vi "Unit Test.vi"() -> ()   [LabVIEW 2018]
uses:
  PPLs/Temp Chamber/Parent/Temp Chamber.lvlibp/Custom Controls/Status.ctl
  PPLs/Temp Chamber/Parent/Temp Chamber.lvlibp/Custom Controls/Profile Status.ctl
  PPLs/Temp Chamber/Parent/Temp Chamber.lvlibp/Custom Controls/Profile State.ctl
  PPLs/Temp Chamber/Parent/Temp Chamber.lvlibp/Custom Controls/Step Status.ctl
  PPLs/Temp Chamber/Parent/Temp Chamber.lvlibp/Custom Controls/Step Type.ctl
  F4T.lvclass
  Custom Controls/Command Data.ctl
  PPLs/Temp Chamber/Parent/Temp Chamber.lvlibp/Temp Chamber.lvclass
  PPLs/Temp Chamber/Parent/Temp Chamber.lvlibp/Custom Controls/Control Mode.ctl
  C:/Projects/LabVIEW/PPLs/Temp Chamber/Parent/Temp Chamber.lvlibp/Temp Chamber.lvclass
panel:
  out "Numeric":i32
  out "Value":dbl
  out "Status 2":T1={"Profile Status"={"Profile State"=enum."Not Running", "Current Profile"=0, "Total Time Remaining"=0, "Total Steps"=0}, "Step Status"={"Current Step"=0, "Step Type"=enum."Instant Change", "Time Remaining"=0}}
  out "Status":T1={"Profile Status"={"Profile State"=enum."Not Running", "Current Profile"=0, "Total Time Remaining"=0, "Total Steps"=0}, "Step Status"={"Current Step"=0, "Step Type"=enum."Instant Change", "Time Remaining"=0}}
  in  "reference":refnum<visa-resource-name>="169.254.242.191"
  out "error out":errorcluster
  in  "error in (no error)":errorcluster
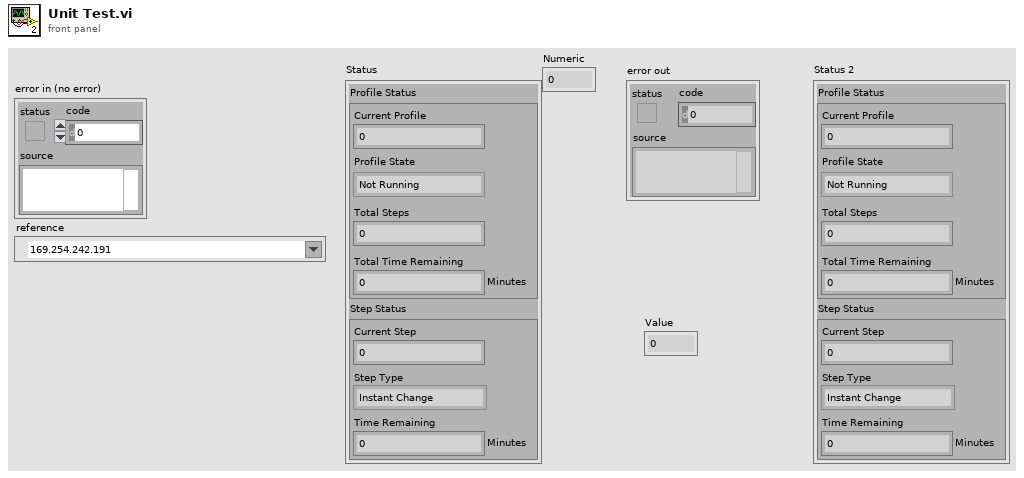
[diagram p1: front panel]
types:
  T1 = typedef "Temp Chamber.lvlibp/Temp Chamber.lvclass/Status.ctl" = cluster{"Profile Status":T2, "Step Status":T4}
  T2 = typedef "Temp Chamber.lvlibp/Temp Chamber.lvclass/Profile Status.ctl" = cluster{"Profile State":T3, "Current Profile":u32, "Total Time Remaining":u32, "Total Steps":u32}
  T3 = typedef "Temp Chamber.lvlibp/Temp Chamber.lvclass/Profile State.ctl" = enum16{"Running", "Not Running", "Paused", "Completed", "Terminated"}
  T4 = typedef "Temp Chamber.lvlibp/Temp Chamber.lvclass/Step Status.ctl" = cluster{"Current Step":u32, "Step Type":T5, "Time Remaining":u32}
  T5 = typedef "Temp Chamber.lvlibp/Temp Chamber.lvclass/Step Type.ctl" = enum16{"Instant Change", "Wait For", "Jump", "Soak", "Ramp Rate", "Ramp Time", "End", "Other"}
  T6 = typedef "F4T.lvlib/F4T.lvclass/Command Data.ctl" = cluster{"ParameterID":u32, "InstanceId":u32, "Value":string}
  T7 = typedef "Temp Chamber.lvlibp/Temp Chamber.lvclass/Control Mode.ctl" = enum16{"Start", "Pause", "Resume", "Stop"}
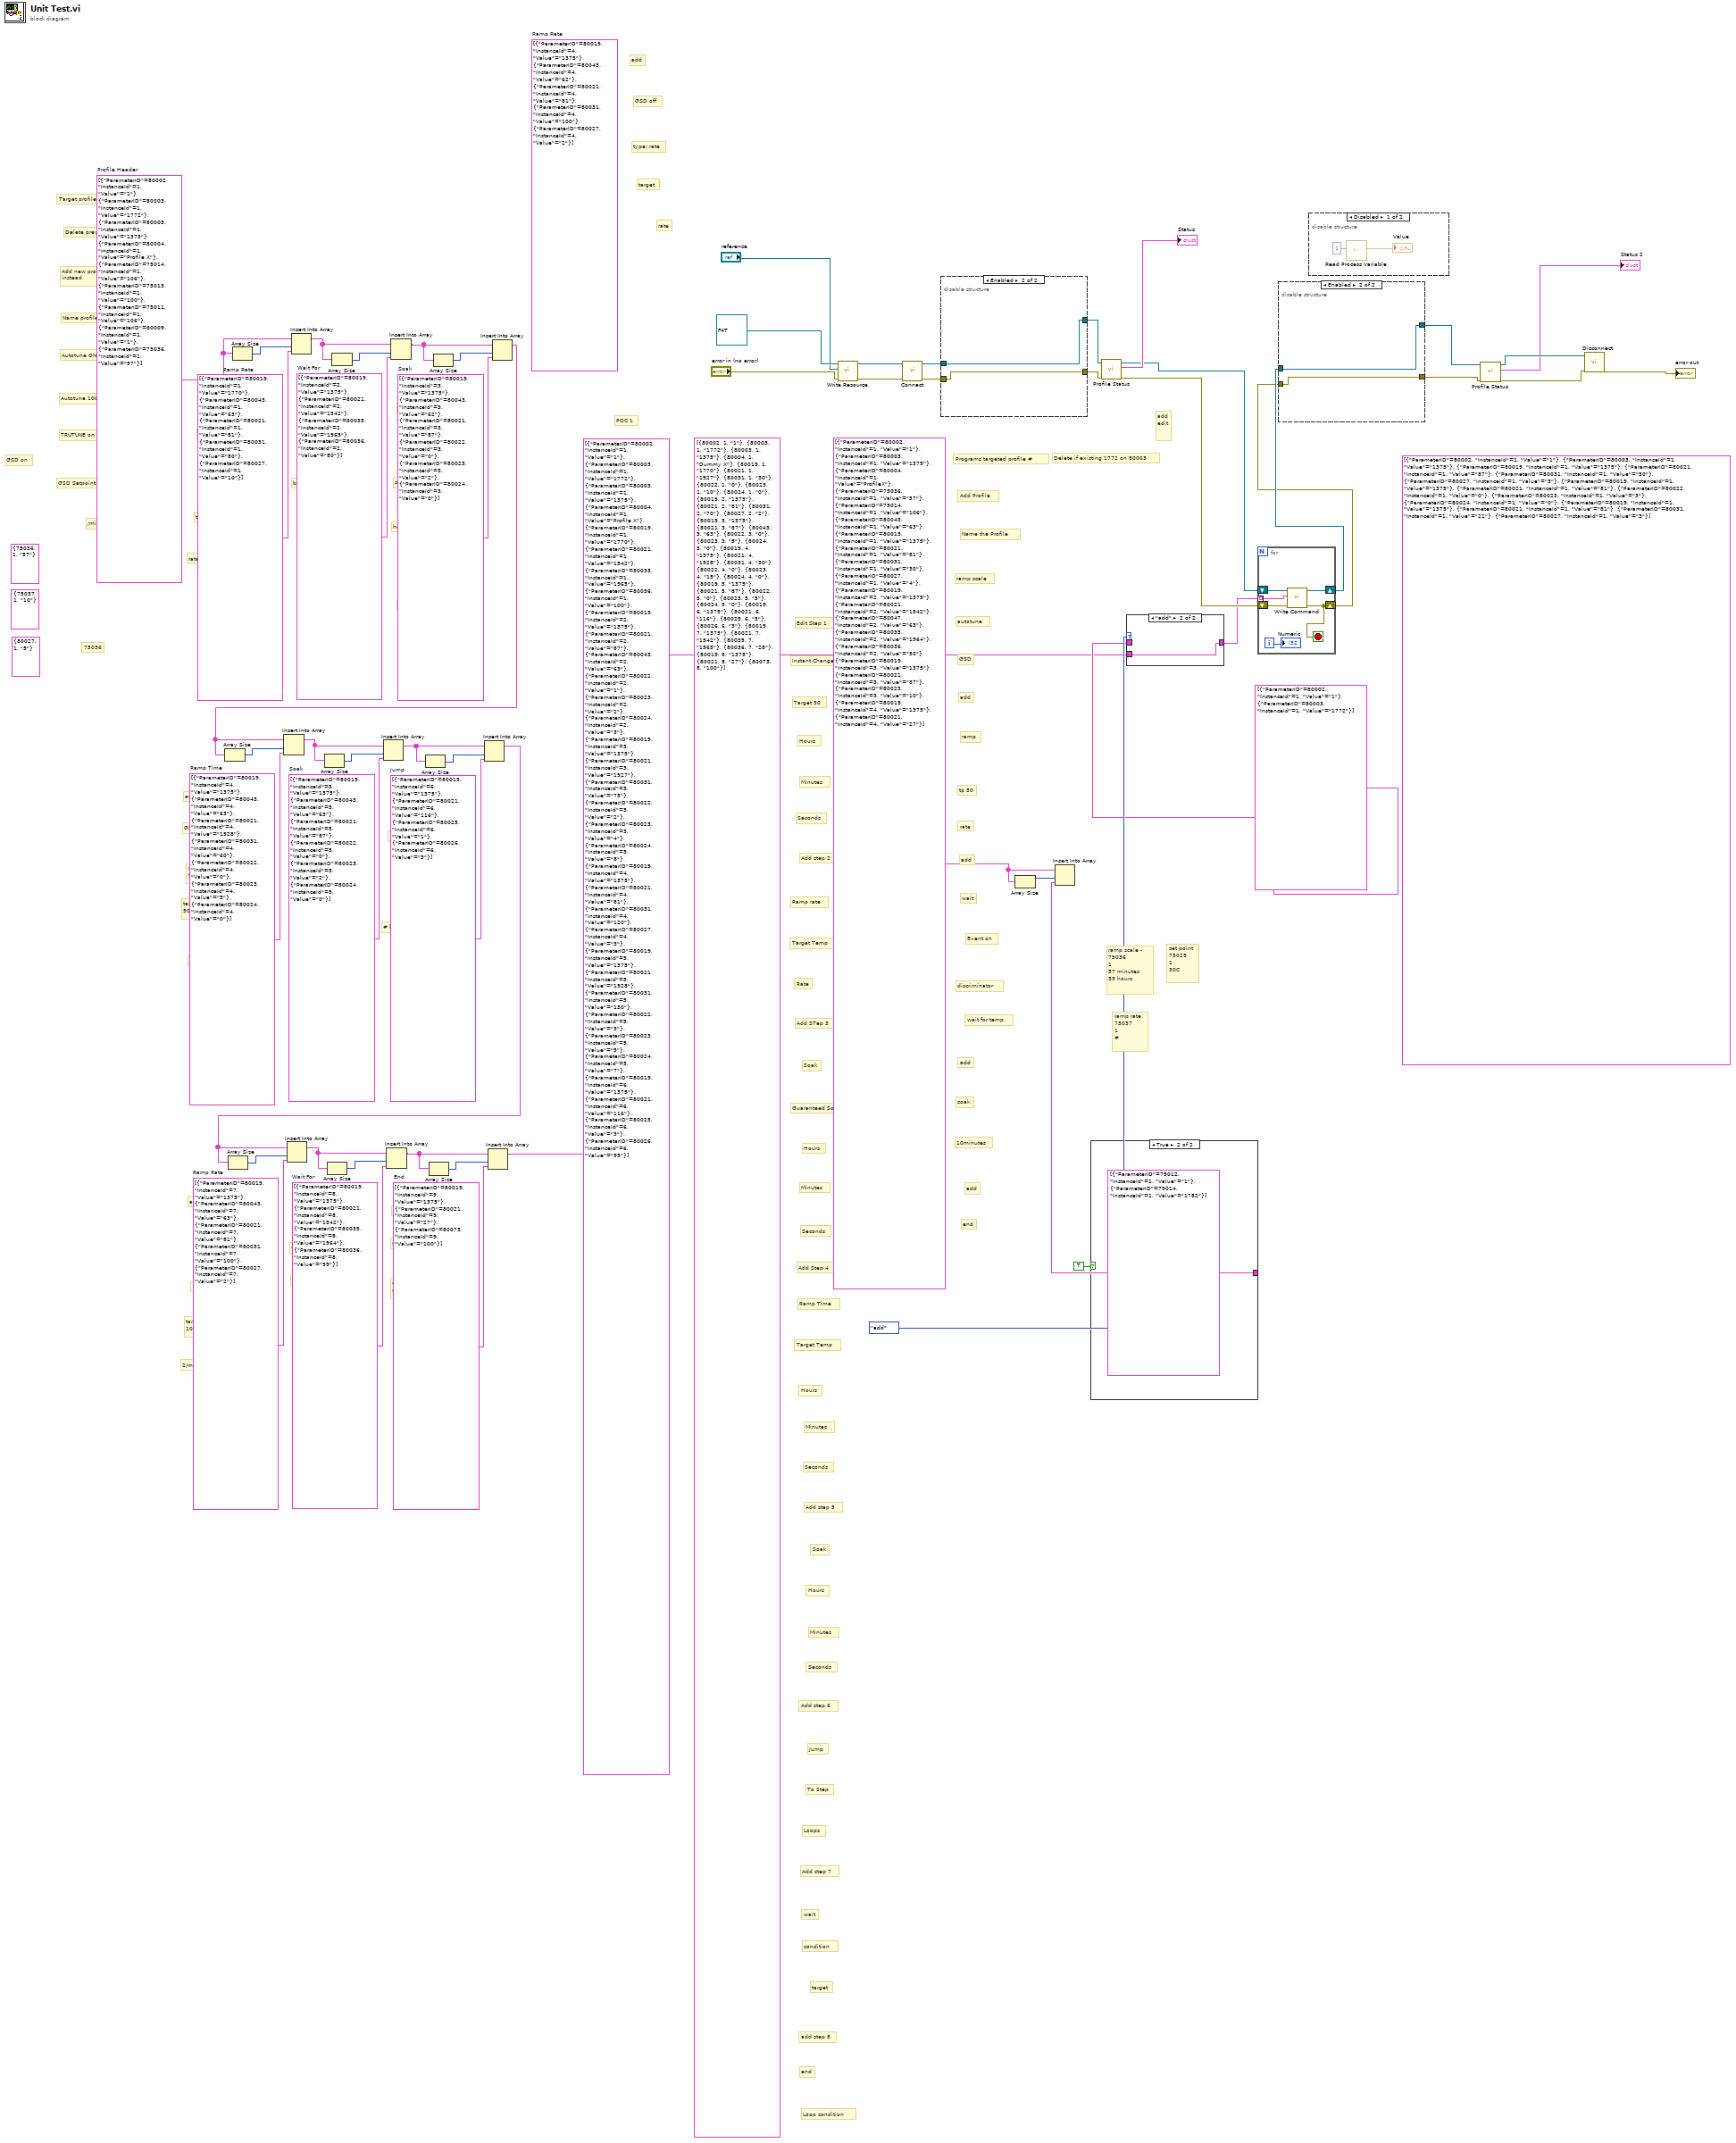
[diagram p0: block diagram]
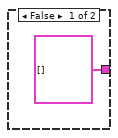
[diagram p2: hidden frame]
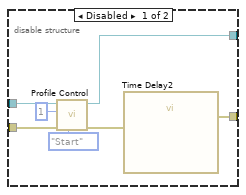
[diagram p4: hidden frame]
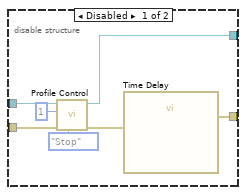
[diagram p6: hidden frame]
diagram:
  (unwired) T6[] [{"ParameterID"=80019, "InstanceId"=4, "Value"="1375"}, {"ParameterID"=80043, "InstanceId"=4, "Value"="62"}, {"ParameterID"=80021, "InstanceId"=4, "Value"="81"}, {"ParameterID"=80031, "InstanceId"=4, "Value"="100"}, {"ParameterID"=80027, "InstanceId"=4, "Value"="2"}]  # Ramp Rate
  (unwired) T6 {"ParameterID"=75036, "InstanceId"=1, "Value"="57"} ("Command Data")
  (unwired) T6 {"ParameterID"=75037, "InstanceId"=1, "Value"="10"} ("Command Data")
  (unwired) T6 {"ParameterID"=80027, "InstanceId"=1, "Value"="5"} ("Command Data")
  w7 = T6[] [{"ParameterID"=80019, "InstanceId"=9, "Value"="1375"}, {"ParameterID"=80021, "InstanceId"=9, "Value"="27"}, {"ParameterID"=80073, "InstanceId"=9, "Value"="100"}]  # End
  w10 = T6[] [{"ParameterID"=80019, "InstanceId"=8, "Value"="1375"}, {"ParameterID"=80021, "InstanceId"=8, "Value"="1542"}, {"ParameterID"=80035, "InstanceId"=8, "Value"="1964"}, {"ParameterID"=80036, "InstanceId"=8, "Value"="99"}]  # Wait For
  w12 = T6[] [{"ParameterID"=80019, "InstanceId"=7, "Value"="1375"}, {"ParameterID"=80043, "InstanceId"=7, "Value"="63"}, {"ParameterID"=80021, "InstanceId"=7, "Value"="81"}, {"ParameterID"=80031, "InstanceId"=7, "Value"="100"}, {"ParameterID"=80027, "InstanceId"=7, "Value"="2"}]  # Ramp Rate
  w15 = T6[] [{"ParameterID"=80019, "InstanceId"=6, "Value"="1375"}, {"ParameterID"=80021, "InstanceId"=6, "Value"="116"}, {"ParameterID"=80025, "InstanceId"=6, "Value"="1"}, {"ParameterID"=80026, "InstanceId"=6, "Value"="3"}]  # Jump
  w18 = T6[] [{"ParameterID"=80019, "InstanceId"=5, "Value"="1375"}, {"ParameterID"=80043, "InstanceId"=5, "Value"="63"}, {"ParameterID"=80021, "InstanceId"=5, "Value"="87"}, {"ParameterID"=80022, "InstanceId"=5, "Value"="0"}, {"ParameterID"=80023, "InstanceId"=5, "Value"="2"}, {"ParameterID"=80024, "InstanceId"=5, "Value"="0"}]  # Soak
  w20 = T6[] [{"ParameterID"=80019, "InstanceId"=4, "Value"="1375"}, {"ParameterID"=80043, "InstanceId"=4, "Value"="63"}, {"ParameterID"=80021, "InstanceId"=4, "Value"="1928"}, {"ParameterID"=80031, "InstanceId"=4, "Value"="60"}, {"ParameterID"=80022, "InstanceId"=4, "Value"="0"}, {"ParameterID"=80023, "InstanceId"=4, "Value"="5"}, {"ParameterID"=80024, "InstanceId"=4, "Value"="0"}]  # Ramp Time
  w22 = T6[] [{"ParameterID"=80019, "InstanceId"=3, "Value"="1375"}, {"ParameterID"=80043, "InstanceId"=3, "Value"="62"}, {"ParameterID"=80021, "InstanceId"=3, "Value"="87"}, {"ParameterID"=80022, "InstanceId"=3, "Value"="0"}, {"ParameterID"=80023, "InstanceId"=3, "Value"="2"}, {"ParameterID"=80024, "InstanceId"=3, "Value"="0"}]  # Soak
  w24 = T6[] [{"ParameterID"=80019, "InstanceId"=2, "Value"="1375"}, {"ParameterID"=80021, "InstanceId"=2, "Value"="1542"}, {"ParameterID"=80035, "InstanceId"=2, "Value"="1965"}, {"ParameterID"=80036, "InstanceId"=2, "Value"="80"}]  # Wait For
  w26 = T6[] [{"ParameterID"=80019, "InstanceId"=1, "Value"="1770"}, {"ParameterID"=80043, "InstanceId"=1, "Value"="63"}, {"ParameterID"=80021, "InstanceId"=1, "Value"="81"}, {"ParameterID"=80031, "InstanceId"=1, "Value"="80"}, {"ParameterID"=80027, "InstanceId"=1, "Value"="10"}]  # Ramp Rate
  w28 = T6[] [{"ParameterID"=80002, "InstanceId"=1, "Value"="1"}, {"ParameterID"=80003, "InstanceId"=1, "Value"="1772"}, {"ParameterID"=80003, "InstanceId"=1, "Value"="1375"}, {"ParameterID"=80004, "InstanceId"=1, "Value"="Profile X"}, {"ParameterID"=75014, "InstanceId"=1, "Value"="106"}, {"ParameterID"=75013, "InstanceId"=1, "Value"="100"}, {"ParameterID"=75011, "InstanceId"=1, "Value"="106"}, {"ParameterID"=80009, "InstanceId"=1, "Value"="1"}, {"ParameterID"=75036, "InstanceId"=1, "Value"="57"}]  # Profile Header
  (unwired) T6[] [{"ParameterID"=80002, "InstanceId"=1, "Value"="1"}, {"ParameterID"=80003, "InstanceId"=1, "Value"="1772"}, {"ParameterID"=80003, "InstanceId"=1, "Value"="1375"}, {"ParameterID"=80004, "InstanceId"=1, "Value"="Dummy X"}, {"ParameterID"=80019, "InstanceId"=1, "Value"="1770"}, {"ParameterID"=80021, "InstanceId"=1, "Value"="1927"}, {"ParameterID"=80031, "InstanceId"=1, "Value"="30"}, {"ParameterID"=80022, "InstanceId"=1, "Value"="0"}, {"ParameterID"=80023, "InstanceId"=1, "Value"="10"}, {"ParameterID"=80024, "InstanceId"=1, "Value"="0"}, {"ParameterID"=80019, "InstanceId"=2, "Value"="1375"}, {"ParameterID"=80021, "InstanceId"=2, "Value"="81"}, {"ParameterID"=80031, "InstanceId"=2, "Value"="70"}, {"ParameterID"=80027, "InstanceId"=2, "Value"="2"}, {"ParameterID"=80019, "InstanceId"=3, "Value"="1375"}, {"ParameterID"=80021, "InstanceId"=3, "Value"="87"}, {"ParameterID"=80043, "InstanceId"=3, "Value"="63"}, {"ParameterID"=80022, "InstanceId"=3, "Value"="0"}, {"ParameterID"=80023, "InstanceId"=3, "Value"="5"}, {"ParameterID"=80024, "InstanceId"=3, "Value"="0"}, {"ParameterID"=80019, "InstanceId"=4, "Value"="1375"}, {"ParameterID"=80021, "InstanceId"=4, "Value"="1928"}, {"ParameterID"=80031, "InstanceId"=4, "Value"="30"}, {"ParameterID"=80022, "InstanceId"=4, "Value"="0"}, {"ParameterID"=80023, "InstanceId"=4, "Value"="15"}, {"ParameterID"=80024, "InstanceId"=4, "Value"="0"}, {"ParameterID"=80019, "InstanceId"=5, "Value"="1375"}, {"ParameterID"=80021, "InstanceId"=5, "Value"="87"}, {"ParameterID"=80022, "InstanceId"=5, "Value"="0"}, {"ParameterID"=80023, "InstanceId"=5, "Value"="5"}, {"ParameterID"=80024, "InstanceId"=5, "Value"="0"}, {"ParameterID"=80019, "InstanceId"=6, "Value"="1375"}, {"ParameterID"=80021, "InstanceId"=6, "Value"="116"}, {"ParameterID"=80025, "InstanceId"=6, "Value"="5"}, {"ParameterID"=80026, "InstanceId"=6, "Value"="3"}, {"ParameterID"=80019, "InstanceId"=7, "Value"="1375"}, {"ParameterID"=80021, "InstanceId"=7, "Value"="1542"}, {"ParameterID"=80035, "InstanceId"=7, "Value"="1965"}, {"ParameterID"=80036, "InstanceId"=7, "Value"="28"}, {"ParameterID"=80019, "InstanceId"=8, "Value"="1375"}, {"ParameterID"=80021, "InstanceId"=8, "Value"="27"}, {"ParameterID"=80073, "InstanceId"=8, "Value"="100"}]
  w32 = T6[] [{"ParameterID"=80002, "InstanceId"=1, "Value"="1"}, {"ParameterID"=80003, "InstanceId"=1, "Value"="1375"}, {"ParameterID"=80004, "InstanceId"=1, "Value"="ProfileX"}, {"ParameterID"=75036, "InstanceId"=1, "Value"="57"}, {"ParameterID"=75014, "InstanceId"=1, "Value"="106"}, {"ParameterID"=80043, "InstanceId"=1, "Value"="63"}, {"ParameterID"=80019, "InstanceId"=1, "Value"="1375"}, {"ParameterID"=80021, "InstanceId"=1, "Value"="81"}, {"ParameterID"=80031, "InstanceId"=1, "Value"="30"}, {"ParameterID"=80027, "InstanceId"=1, "Value"="4"}, {"ParameterID"=80019, "InstanceId"=2, "Value"="1375"}, {"ParameterID"=80021, "InstanceId"=2, "Value"="1542"}, {"ParameterID"=80047, "InstanceId"=2, "Value"="63"}, {"ParameterID"=80035, "InstanceId"=2, "Value"="1964"}, {"ParameterID"=80036, "InstanceId"=2, "Value"="50"}, {"ParameterID"=80019, "InstanceId"=3, "Value"="1375"}, {"ParameterID"=80021, "InstanceId"=3, "Value"="87"}, {"ParameterID"=80023, "InstanceId"=3, "Value"="10"}, {"ParameterID"=80019, "InstanceId"=4, "Value"="1375"}, {"ParameterID"=80021, "InstanceId"=4, "Value"="27"}]
  (unwired) T6[] [{"ParameterID"=80002, "InstanceId"=1, "Value"="1"}, {"ParameterID"=80003, "InstanceId"=1, "Value"="1375"}, {"ParameterID"=80019, "InstanceId"=1, "Value"="1375"}, {"ParameterID"=80021, "InstanceId"=1, "Value"="87"}, {"ParameterID"=80031, "InstanceId"=1, "Value"="50"}, {"ParameterID"=80027, "InstanceId"=1, "Value"="3"}, {"ParameterID"=80019, "InstanceId"=1, "Value"="1375"}, {"ParameterID"=80021, "InstanceId"=1, "Value"="81"}, {"ParameterID"=80022, "InstanceId"=1, "Value"="0"}, {"ParameterID"=80023, "InstanceId"=1, "Value"="3"}, {"ParameterID"=80024, "InstanceId"=1, "Value"="0"}, {"ParameterID"=80019, "InstanceId"=1, "Value"="1375"}, {"ParameterID"=80021, "InstanceId"=1, "Value"="81"}, {"ParameterID"=80031, "InstanceId"=1, "Value"="21"}, {"ParameterID"=80027, "InstanceId"=1, "Value"="3"}]
  (unwired) T6[] [{"ParameterID"=80002, "InstanceId"=1, "Value"="1"}, {"ParameterID"=80003, "InstanceId"=1, "Value"="1772"}, {"ParameterID"=80003, "InstanceId"=1, "Value"="1375"}, {"ParameterID"=80004, "InstanceId"=1, "Value"="Profile X"}, {"ParameterID"=80019, "InstanceId"=1, "Value"="1770"}, {"ParameterID"=80021, "InstanceId"=1, "Value"="1542"}, {"ParameterID"=80035, "InstanceId"=1, "Value"="1965"}, {"ParameterID"=80036, "InstanceId"=1, "Value"="100"}, {"ParameterID"=80019, "InstanceId"=2, "Value"="1375"}, {"ParameterID"=80021, "InstanceId"=2, "Value"="87"}, {"ParameterID"=80043, "InstanceId"=2, "Value"="63"}, {"ParameterID"=80022, "InstanceId"=2, "Value"="1"}, {"ParameterID"=80023, "InstanceId"=2, "Value"="2"}, {"ParameterID"=80024, "InstanceId"=2, "Value"="3"}, {"ParameterID"=80019, "InstanceId"=3, "Value"="1375"}, {"ParameterID"=80021, "InstanceId"=3, "Value"="1927"}, {"ParameterID"=80031, "InstanceId"=3, "Value"="75"}, {"ParameterID"=80022, "InstanceId"=3, "Value"="2"}, {"ParameterID"=80023, "InstanceId"=3, "Value"="4"}, {"ParameterID"=80024, "InstanceId"=3, "Value"="8"}, {"ParameterID"=80019, "InstanceId"=4, "Value"="1375"}, {"ParameterID"=80021, "InstanceId"=4, "Value"="81"}, {"ParameterID"=80031, "InstanceId"=4, "Value"="120"}, {"ParameterID"=80027, "InstanceId"=4, "Value"="3"}, {"ParameterID"=80019, "InstanceId"=5, "Value"="1375"}, {"ParameterID"=80021, "InstanceId"=5, "Value"="1928"}, {"ParameterID"=80031, "InstanceId"=5, "Value"="130"}, {"ParameterID"=80022, "InstanceId"=5, "Value"="3"}, {"ParameterID"=80023, "InstanceId"=5, "Value"="5"}, {"ParameterID"=80024, "InstanceId"=5, "Value"="7"}, {"ParameterID"=80019, "InstanceId"=6, "Value"="1375"}, {"ParameterID"=80021, "InstanceId"=6, "Value"="116"}, {"ParameterID"=80025, "InstanceId"=6, "Value"="3"}, {"ParameterID"=80026, "InstanceId"=6, "Value"="95"}]
  # "GSD"
  # "GSD"
  # "GSD"
  # "GSD"
  # "GSD"
  # "rate"
  # "target"
  # "type: rate"
  # "GSD off"
  # "add"
  # "GSD Setpoint"
  # "/min"
  # "75036"
  # "2/min?"
  # "target\n100"
  # "rate"
  # "add"
  # "rate 10"
  # "to 80"
  # "rate"
  # "edit"
  # "sec"
  # "min"
  # "hrs"
  # "target\n50"
  # "ramp\ntime"
  # "add"
  # "99"
  # "above"
  # "wait"
  # "add"
  # "# loops"
  # "to\nstep"
  # "jump"
  # "add"
  # "sec"
  # "min"
  # "hrs"
  # "soak"
  # "add"
  # "user\nctrl"
  # "end"
  # "add"
  # "secs"
  # "mins"
  # "hours"
  # "soak"
  # "add"
  # "80"
  # "below"
  # "Wait"
  # "add"
  # "GSD on"
  # "TRUTUNE on"
  # "Autotune 100%"
  # "Autotune ON"
  # "Name profile"
  # "Add new profile\ninstead"
  # "Delete previous"
  # "Target profile"
  # "Loop condition"
  # "end"
  # "add step 8"
  # "target"
  # "condition"
  # "wait"
  # "Add step 7"
  # "Loops"
  # "To Step"
  # "Jump"
  # "Add step 6"
  # "Seconds"
  # "Minutes"
  # "Hours"
  # "Soak"
  # "Add step 5"
  # "Seconds"
  # "Minutes"
  # "Hours"
  # "Target Temp"
  # "Ramp Time"
  # "Add Step 4"
  # "Seconds"
  # "Minutes"
  # "Hours"
  # "Guaranteed Soak"
  # "Soak"
  # "Add STep 3"
  # "Rate"
  # "Target Temp"
  # "Ramp rate"
  # "Add step 2"
  # "Seconds"
  # "Minutes"
  # "Hours"
  # "Target 30"
  # "Instant Change"
  # "Edit Step 1"
  # "POC 1"
  # "Name the Profile"
  # "Add Profile"
  # "Delete if existing 1772 on 80003"
  # "Programs targeted profile #"
  # "Event on"
  # "wait for temp"
  # "discriminator"
  # "wait"
  # "add"
  # "ramp scale"
  # "ramp rate\n75037\n1\n#"
  # "set point\n75029\n1\n30C"
  # "ramp scale - \n75036\n1\n57 minutes\n39 hours"
  # "10minutes"
  # "soak"
  # "add"
  # "autotune"
  # "end"
  # "add"
  # "rate"
  # "tp 50"
  # "ramp"
  # "add"
  # "GSD"
  # "add\nedit"
  n1 = Array Size(array=w28) -> (size(s)=w27:i32)
  n2 = Insert Into Array(array=w28, index=w27, new element=w26) -> (w4:T6[])
  n3 = Array Size(array=w4) -> (size(s)=w25:i32)
  n4 = Insert Into Array(array=w4, index=w25, new element=w24) -> (w3:T6[])
  n5 = Array Size(array=w3) -> (size(s)=w23:i32)
  n6 = Insert Into Array(array=w3, index=w23, new element=w22) -> (w2:T6[])
  n7 = Array Size(array=w2) -> (size(s)=w21:i32)
  n8 = Insert Into Array(array=w2, index=w21, new element=w20) -> (w17:T6[])
  n9 = Array Size(array=w17) -> (size(s)=w19:i32)
  n10 = Insert Into Array(array=w17, index=w19, new element=w18) -> (w14:T6[])
  n11 = Array Size(array=w14) -> (size(s)=w16:i32)
  n12 = Insert Into Array(array=w14, index=w16, new element=w15) -> (w5:T6[])
  n13 = Array Size(array=w5) -> (size(s)=w13:i32)
  n14 = Insert Into Array(array=w5, index=w13, new element=w12) -> (w9:T6[])
  n15 = Array Size(array=w9) -> (size(s)=w11:i32)
  n16 = Insert Into Array(array=w9, index=w11, new element=w10) -> (w6:T6[])
  n17 = Array Size(array=w6) -> (size(s)=w8:i32)
  n18 = Insert Into Array(array=w6, index=w8, new element=w7) -> (w1:T6[])
  n19 = call "Write Resource.vi"("error in (no error)"="error in (no error)", "Resource"="reference", "Temp Chamber in"=refnum<class "F4T.lvclass"> refnum ("F4T.lvlib:F4T.lvclass")) -> ("error out"=w51:errorcluster, "Temp Chamber out"=w52:refnum<class "F4T.lvclass">)  [unwired: 7 in]
  n20 = call-dynamic "Connect.vi"("error in (no error)"=w51, "F4T in"=w52) -> ("error out"=w49:errorcluster, "F4T out"=w50:refnum<class "F4T.lvclass">)  [unwired: 8 in]
  n21 = disable-structure shown="Enabled" {
    disable-tunnel: w50 -> [w62 w64]
    disable-tunnel: w49 -> [w61 w63]
    disable-tunnel: [w57 w64] -> w47
    disable-tunnel: [w56 w63] -> w46
    frame Disabled {
      n22 = call-dynamic "Profile Control.vi"("Control Mode"=Control_Mode."Stop", "error in (no error)"=w61, "Profile Number"=u32 1, "F4T in"=w62) -> ("error out"=w58:errorcluster, "F4T out"=w57:refnum<class "F4T.lvclass">)  [unwired: 6 in]
      n23 = call "Time Delay"("error in (no error)"=w58) -> ("error out"=w56:errorcluster)  [unwired: 10 in]
    }
    frame Enabled {
    }
  }
  n24 = Array Size(array=w32) -> (size(s)=w31:i32)
  n25 = case shown="True" TRUE {
    tunnel: [T6[] [] T6[] [{"ParameterID"=79012, "InstanceId"=1, "Value"="1"}, {"ParameterID"=79014, "InstanceId"=1, "Value"="1782"}]] -> w30
    frame False {
    }
    frame True {
    }
  }
  n26 = Insert Into Array(array=w32, index=w31, new element=w30) -> ()  [unwired: 1 out]
  n27 = call-dynamic "Profile Status.vi"("error in (no error)"=w46, "F4T in"=w47) -> ("error out"=w40:errorcluster, "Status"=→"Status":T1, "F4T out"=w41:refnum<class "F4T.lvclass">)  [unwired: 7 in]
  n28 = case shown="\"add\"" enum16{"delete", "add"}."add" {
    tunnel: T6[] [{"ParameterID"=80002, "InstanceId"=1, "Value"="1"}, {"ParameterID"=80003, "InstanceId"=1, "Value"="1772"}] -> [w67 _]
    tunnel: [w67 w68] -> w33
    tunnel: w1 -> [_ w68]
    frame "delete", Default {
    }
    frame "add" {
    }
  }
  n29 = for {
    shift-right: [w73] -> w38
    shift-left: w41 -> [w74]
    tunnel: w33 -> [w72] mode=indexing
    shift-right: [w70] -> w37
    shift-left: w40 -> [w71]
    i -> [w69]
    stop <- w70 stop-if-true
    n30 = call "Write Command.vi"("error in (no error)"=w71, "Command Data"=w72, "F4T in"=w74) -> ("error out"=w70:errorcluster, "F4T out"=w73:refnum<class "F4T.lvclass">)  [unwired: 7 in]
    "Numeric" <- w69
  }
  n31 = disable-structure shown="Enabled" {
    disable-tunnel: w38 -> [w81 w83]
    disable-tunnel: w37 -> [w80 w82]
    disable-tunnel: [w76 w83] -> w36
    disable-tunnel: [w75 w82] -> w35
    frame Disabled {
      n32 = call-dynamic "Profile Control.vi"("Control Mode"=Control_Mode."Start", "error in (no error)"=w80, "Profile Number"=u32 1, "F4T in"=w81) -> ("error out"=w77:errorcluster, "F4T out"=w76:refnum<class "F4T.lvclass">)  [unwired: 6 in]
      n33 = call "Time Delay2"("error in (no error)"=w77) -> ("error out"=w75:errorcluster)  [unwired: 10 in]
    }
    frame Enabled {
    }
  }
  n34 = disable-structure shown="Disabled" {
    frame Disabled {
      n35 = call-dynamic "Read Process Variable.vi"("Process Variable"=u32 1) -> ("Value"=→"Value":dbl)  [unwired: 8 in, 2 out]
    }
    frame Enabled {
    }
  }
  n36 = call-dynamic "Profile Status.vi"("error in (no error)"=w35, "F4T in"=w36) -> ("error out"=w43:errorcluster, "Status"=→"Status 2":T1, "F4T out"=w45:refnum<class "F4T.lvclass">)  [unwired: 7 in]
  n37 = call-dynamic "Disconnect.vi"("error in (no error)"=w43, "F4T in"=w45) -> ("error out"=→"error out":errorcluster)  [unwired: 8 in, 1 out]
